vi "Main.vi"() -> ()   [LabVIEW 2019]
panel:
  out "T1":waveform(dbl)[](graph)
  out "T0":waveform(dbl)[](graph)
  in  "Readout Interval (ms)":i32=1000
  in  "units":i32(ring) items=["degC", "degF", "kelvin", "raw"]
  in  "Device/Channel Name":string="Dev0/Ti0:1"
  out "error out":errorcluster={"status"=TRUE, "code"=0, "source"=""}
  out "T1":dbl
  out "T0":dbl
  out "Readout Status":bool
  out "Init. Status":bool=TRUE
  out "Last Measured":timestamp format="%<%Y-%m-%d %H:%M:%S>T"
  in  "Stop":bool
  # "Thermocouples for Manual Annealing Control System"
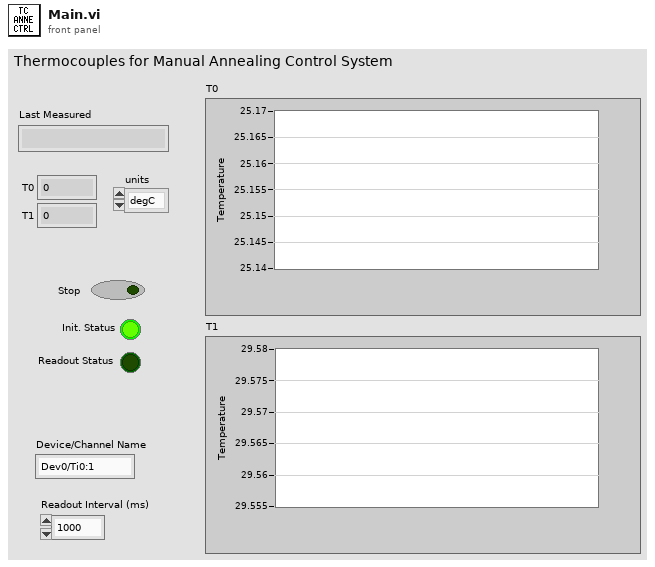
[diagram p1: front panel]
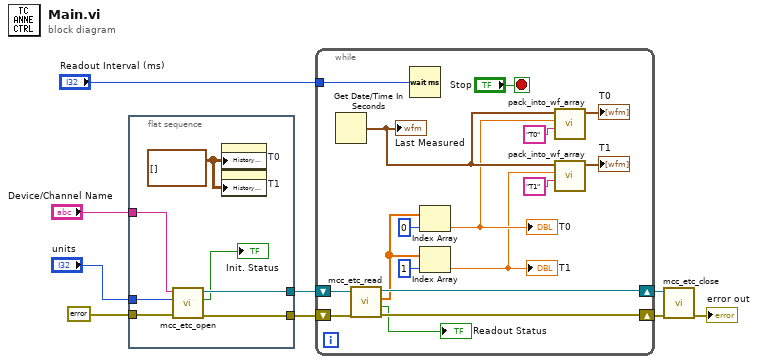
[diagram p0: block diagram]
diagram:
  n1 = flat-sequence {
    tunnel: [w16] -> w9
    tunnel: errorcluster {"status"=FALSE, "code"=0, "source"=""} ("error in") -> [w15]
    tunnel: [w14] -> w7
    tunnel: "Device/Channel Name" -> [w12]
    tunnel: "units" -> [w11]
    frame #0 {
      w10 = waveform(dbl)[][] [] ("History Data")
      n2 = call "mcc_etc_open.vi"("error in"=w15, "units"=w11, "name"=w12) -> ("error out"=w14:errorcluster, "status"=→"Init. Status":bool, "task out"=w16:refnum<k24>)  [unwired: 6 in]
      n3 = property on="T0" class="WFChart (strict)"("History Data"=w10) -> ()  [unwired: 2 in, 2 out]
      n4 = property on="T1" class="WFChart (strict)"("History Data"=w10) -> ()  [unwired: 2 in, 2 out]
    }
  }
  n5 = while {
    shift-right: [w27] -> w5
    shift-left: w7 -> [w28]
    shift-right: [w26] -> w6
    shift-left: w9 -> [w31]
    tunnel: "Readout Interval (ms)" -> [w22]
    stop <- "Stop" stop-if-true
    n6 = Get Date/Time In Seconds() -> (seconds since 1Jan1904=w32:timestamp)
    "Last Measured" <- w32
    n7 = call "mcc_etc_read.vi"("error in"=w28, "task in"=w31) -> ("error out"=w27:errorcluster, "status"=→"Readout Status":bool, "temperature_array"=w24:dbl[], "task out"=w26:refnum<k24>)  [unwired: 6 in]
    n8 = Wait (ms)(milliseconds to wait=w22) -> ()  [unwired: 1 out]
    n9 = Index Array(array=w24, index=0) -> (element=w23:dbl)
    "T0" <- w23
    n10 = Index Array(array=w24, index=1) -> (element=w17:dbl)
    "T1" <- w17
    n11 = call "pack_into_wf_array.vi"("name"="T0", "value"=w23, "time"=w32) -> ("waveform_array"=→"T0":waveform(dbl)[])  [unwired: 8 in]
    n12 = call "pack_into_wf_array.vi"("name"="T1", "value"=w17, "time"=w32) -> ("waveform_array"=→"T1":waveform(dbl)[])  [unwired: 8 in]
  }
  n13 = call "mcc_etc_close.vi"("error in"=w5, "task in"=w6) -> ("error out"=→"error out":errorcluster)  [unwired: 8 in, 1 out]
